vi "Read background.vi"(8 "error in (no error)":errorcluster, 11 "_camera in":refnum<class "_camera.lvclass">) -> (0 "error out":errorcluster, 2 "background":i32[][](array[numeric]), 3 "_camera out":refnum<class "_camera.lvclass">)   [LabVIEW 2019, in "_camera.lvlib" / "_camera.lvclass"]
uses:
  _camera.lvclass
  _camera.lvclass/_camera.ctl
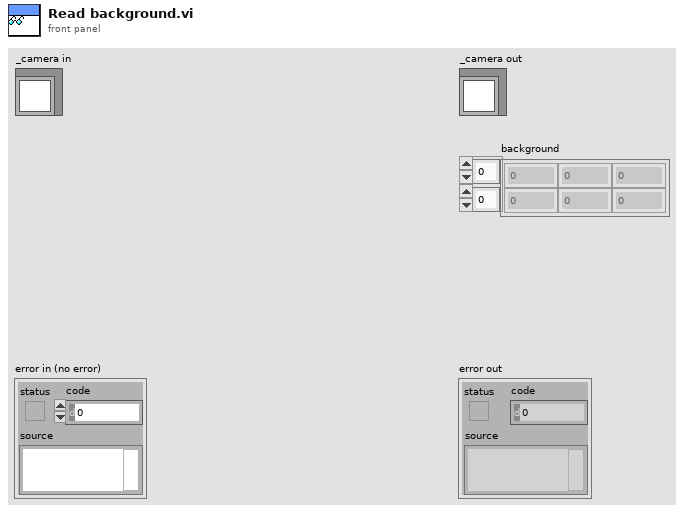
[diagram p1: front panel]
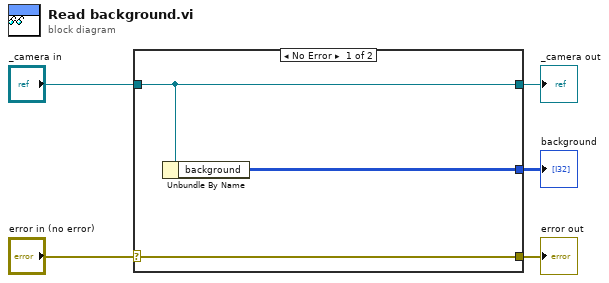
[diagram p0: block diagram]
diagram:
  n1 = case shown="No Error" "error in (no error)" {
    selector: "error in (no error)" -> [w8 w9]
    tunnel: [w8 w9] -> w4
    tunnel: [w7 w10] -> w2
    tunnel: "_camera in" -> [w7 w10]
    tunnel: [w6 _] -> w1
    frame No Error {
      n2 = Unbundle By Name(w7) -> ("background"=w6:i32[][])
    }
    frame Error {
    }
  }
  "error out" <- w4
  "_camera out" <- w2
  "background" <- w1
